vi "runLT_img.vi"   [LabVIEW 2015]
uses:
  phlib.dll
types:
  T1 = cluster{"initialized":bool, "devidx":i32, "Ch0 Level":i32, "Ch0 ZeroX":i32, "Ch1 Level":i32, "Ch1 ZeroX":i32, "sync rate":i32, "resolution":i32, "acq time":i32, "acq rate":i32, "# bins":u32, "Bin size":enum16{"1", "2", "4", "8", "16", "32", "64", "128"}, "min photons":u32, "truncate":u32}
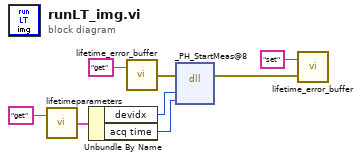
[diagram p0: block diagram]
diagram:
  n1 = call "lifetimeparameters.vi"("command"="get") -> ("Params out"=w5:T1)  [unwired: 1 in]
  n2 = Unbundle By Name(w5) -> ("devidx"=w7:i32, "acq time"=w6:i32)
  n3 = call "lifetime_error_buffer.vi"("command"="get") -> ("error out"=w3:errorcluster)  [unwired: 1 in]
  n4 = dll-call lib="phlib.dll" fn="_PH_StartMeas@8" label="PH_StartMeas"(error in=w3, "devidx"=w7, "tacq"=w6) -> (error out=w1:errorcluster)  [unwired: 5 in, 1 out]
  n5 = call "lifetime_error_buffer.vi"("error in"=w1, "command"="set") -> ()  [unwired: 1 out]
